vi "RTS Client Volt Freq Command Send.vi"(7 "Station":u16=1 min=1 max=8 step=1, 8 "Error In":errorcluster, 9 "Voltage":dbl, 10 "Frequency":T3 items=["60 Hz", "50 Hz"], 11 "Wh Reset":T2) -> (0 "Error Out":errorcluster, 3 "Output Command":string)   [LabVIEW 2020]
uses:
  Type Definitions/RTS Frequency Selector.ctl
  Type Definitions/RTS Reset Watt Hours.ctl
  Type Definitions/RTS Custom Commands.ctl
panel:
  in  "Custom CMD 3":T1="RstWh-"
  in  "Custom CMD 2":T1="Freq-"
  in  "Custom CMD":T1="Volt-"
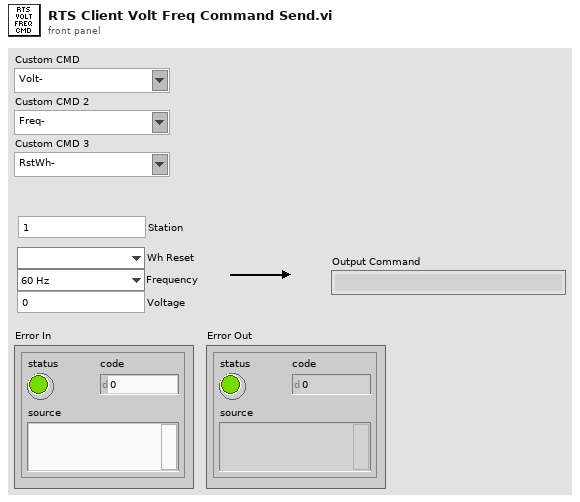
[diagram p1: front panel]
types:
  T1 = typedef "RTS Custom Commands.ctl" = string
  T2 = typedef "RTS Reset Watt Hours.ctl" = enum16{"", "Reset Watt Hours"}
  T3 = typedef "RTS Frequency Selector.ctl" = u16
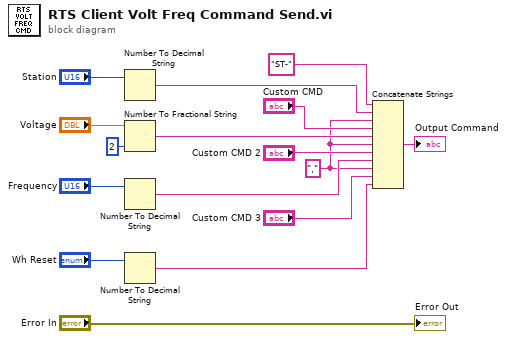
[diagram p0: block diagram]
diagram:
  w1 = "," ("string")
  n1 = Number To Decimal String(number="Station") -> (decimal integer string=w2:string)  [unwired: 1 in]
  n2 = Number To Fractional String(number="Voltage", precision (6)=i16 2) -> (F-format string=w15:string)  [unwired: 2 in]
  n3 = Number To Decimal String(number="Frequency") -> (decimal integer string=w8:string)  [unwired: 1 in]
  n4 = Number To Decimal String(number="Wh Reset") -> (decimal integer string=w6:string)  [unwired: 1 in]
  n5 = Concatenate Strings("ST-" ("string"), w2, w1, "Custom CMD", w15, w1, "Custom CMD 2", w8, w1, "Custom CMD 3", w6) -> (→"Output Command":string)
  "Error Out" <- "Error In"
